vi "Init_Variables.vi"(2 "error in":errorcluster, 3 "task in":refnum<class "Visualization.lvclass">) -> (0 "error out":errorcluster, 1 "task out":refnum<class "Visualization.lvclass">)   [LabVIEW 2018]
uses:
  <vilib>/Quanser/Rapid Control Prototyping Toolkit/visualization/Visualization.lvclass
  <vilib>/Quanser/Rapid Control Prototyping Toolkit/visualization/Visualization Select Variable (1D SGL).vi
  <vilib>/Quanser/Rapid Control Prototyping Toolkit/visualization/Visualization Select Variable (2D SGL).vi
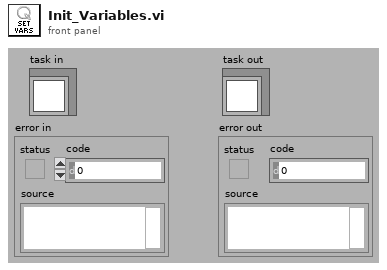
[diagram p1: front panel]
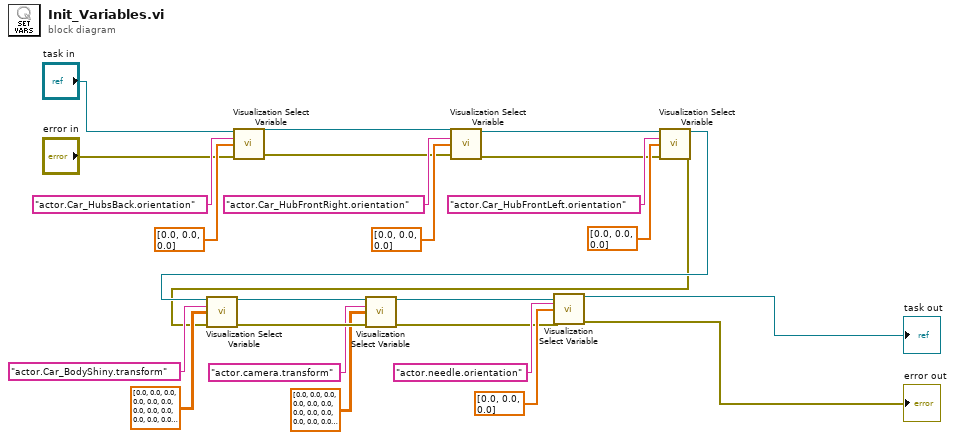
[diagram p0: block diagram]
diagram:
  n1 = call-poly <vilib>:"Visualization Select Variable.vi"("visualization in"="task in", "variable name"="actor.Car_HubsBack.orientation", "initial values"=sgl[] [0.0, 0.0, 0.0] ("initial value"), "error in (no error)"="error in") -> ("visualization out"=w14:refnum<class "Visualization.lvclass">, "error out"=w17:errorcluster)  [unwired: 10 in]
  n2 = call-poly <vilib>:"Visualization Select Variable.vi"("visualization in"=w14, "variable name"="actor.Car_HubFrontRight.orientation", "initial values"=sgl[] [0.0, 0.0, 0.0] ("initial value"), "error in (no error)"=w17) -> ("visualization out"=w13:refnum<class "Visualization.lvclass">, "error out"=w16:errorcluster)  [unwired: 10 in]
  n3 = call-poly <vilib>:"Visualization Select Variable.vi"("visualization in"=w13, "variable name"="actor.Car_HubFrontLeft.orientation", "initial values"=sgl[] [0.0, 0.0, 0.0] ("initial value"), "error in (no error)"=w16) -> ("visualization out"=w8:refnum<class "Visualization.lvclass">, "error out"=w7:errorcluster)  [unwired: 10 in]
  n4 = call-poly <vilib>:"Visualization Select Variable.vi"("visualization in"=w8, "variable name"="actor.Car_BodyShiny.transform", "initial values"=sgl[][] [[0.0, 0.0, 0.0, 0.0], [0.0, 0.0, 0.0, 0.0], [0.0, 0.0, 0.0, 0.0], [0.0, 0.0, 0.0, 0.0]] ("initial value"), "error in (no error)"=w7) -> ("visualization out"=w5:refnum<class "Visualization.lvclass">, "error out"=w6:errorcluster)  [unwired: 10 in]
  n5 = call-poly <vilib>:"Visualization Select Variable.vi"("visualization in"=w5, "variable name"="actor.camera.transform", "initial values"=sgl[][] [[0.0, 0.0, 0.0, 0.0], [0.0, 0.0, 0.0, 0.0], [0.0, 0.0, 0.0, 0.0], [0.0, 0.0, 0.0, 0.0]] ("initial value"), "error in (no error)"=w6) -> ("visualization out"=w2:refnum<class "Visualization.lvclass">, "error out"=w1:errorcluster)  [unwired: 10 in]
  n6 = call-poly <vilib>:"Visualization Select Variable.vi"("visualization in"=w2, "variable name"="actor.needle.orientation", "initial values"=sgl[] [0.0, 0.0, 0.0] ("initial value"), "error in (no error)"=w1) -> ("visualization out"=→"task out":refnum<class "Visualization.lvclass">, "error out"=→"error out":errorcluster)  [unwired: 10 in]
